vi "Append SDI.vi"(8 "error in":errorcluster, 9 "sdi value":u8, 10 "sdi enabled":bool, 11 "configuration string":string) -> (0 "error out":errorcluster, 3 "configuration string out":string)   [LabVIEW 2020, in "Ballard ARINC 429 Hardware Configuration.lvlib"]
uses:
  Ballard ARINC 429 Hardware Configuration.lvlib
  Constants.vi
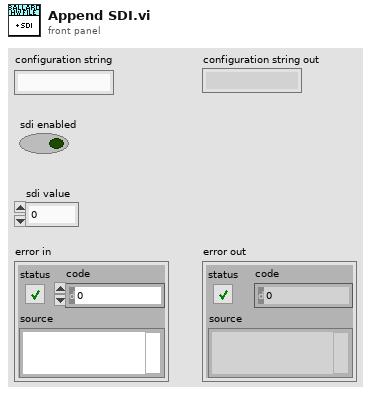
[diagram p1: front panel]
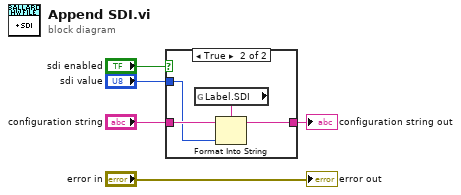
[diagram p0: block diagram]
diagram:
  n1 = case shown="True" "sdi enabled" {
    tunnel: "configuration string" -> [w6 w10]
    tunnel: "sdi value" -> [_ w8]
    tunnel: [w6 w7] -> w4
    frame False {
    }
    frame True {
      n2 = global read "Constants.vi" "Label.SDI"() -> (w9:string)
      n3 = Format Into String(format string=w9, initial string=w10, w8) -> (resulting string=w7:string)  [unwired: 1 in, 1 out]
    }
  }
  "configuration string out" <- w4
  "error out" <- "error in"
